vi "Write String.vi"(8 "error in (no error)":errorcluster, 10 "String":string, 11 "Serial in":refnum<class "Serial.lvclass">) -> (0 "error out":errorcluster, 3 "Serial out":refnum<class "Serial.lvclass">)   [LabVIEW 2024, in "Serial.lvclass"]
doc: "Serial.lvclass:Write String.vi\n\nThis VI is used to write strings (commands, data requests) to the serial port.\n\nInstrument Communication Module Version 1.0\nAugust, 2017 Original Code Consulting David Thomson\n www.originalcode.com"
uses:
  Serial.lvclass
  Serial.lvclass/Serial.ctl
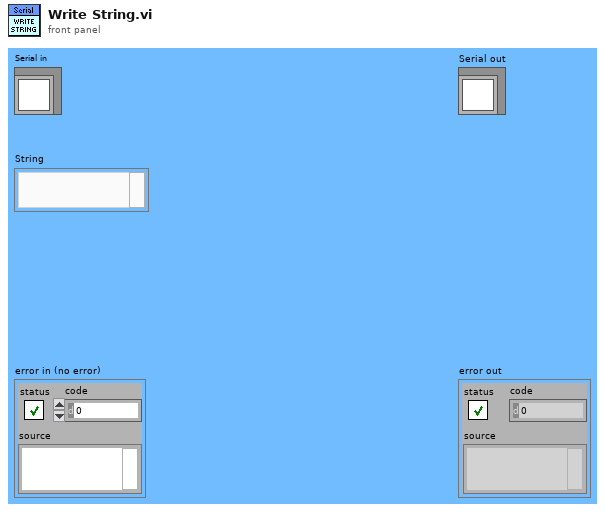
[diagram p1: front panel]
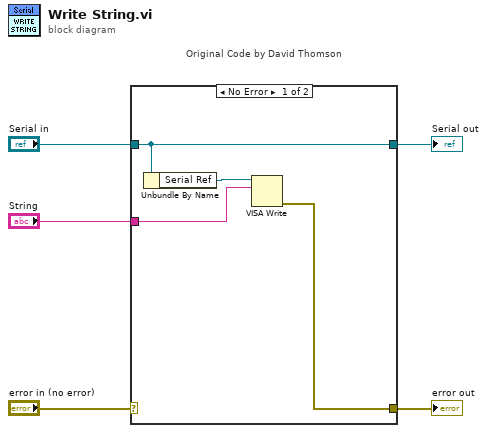
[diagram p0: block diagram]
diagram:
  n1 = case "Original Code by David Thomson" shown="No Error" "error in (no error)" {
    selector: "error in (no error)" -> [_ w11]
    tunnel: [w6 w11] -> w4
    tunnel: [w9 w10] -> w2
    tunnel: "Serial in" -> [w9 w10]
    tunnel: "String" -> [w7 _]
    frame No Error {
      n2 = Unbundle By Name(w9) -> ("Serial Ref"=w8:refnum<visa-resource-name>)
      n3 = VISA Write(VISA resource name=w8, write buffer=w7) -> (error out=w6:errorcluster)  [unwired: 1 in, 2 out]
    }
    frame Error {
    }
  }
  "error out" <- w4
  "Serial out" <- w2
